vi "First Char.vi"(10 "String in":string) -> (1 "First Char":string, 2 "String":string)   [LabVIEW 2020, in "Library Commun.lvlib" / "JSON Value.lvclass"]
doc: "Returns first character from string."
uses:
  JSON Value.lvclass
  <vilib>/Utility/error.llb/whitespace.ctl
  JSON Scalar/JSON Scalar.lvclass
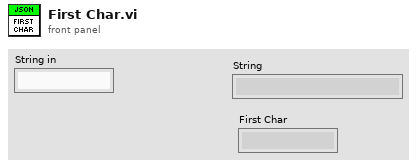
[diagram p1: front panel]
types:
  T1 = typedef "whitespace.ctl" = u16
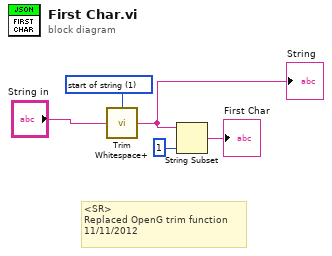
[diagram p0: block diagram]
diagram:
  w1 = T1 1 items=["both", "start of string", "end of string"] ("location (both)")
  # "<SR>\nReplaced OpenG trim function\n11/11/2012"
  n1 = call "Trim Whitespace+.vi"("String"="String in", "location (both)"=w1) -> ("Trimmed String"=w2:string)
  "String" <- w2
  n2 = String Subset(string=w2, length (rest)=1 ("length (rest)")) -> (substring=→"First Char":string)  [unwired: 1 in]
